vi "Channel_selector.vi"(11 "EEG_Data(all_Ch)":dbl[][](array[numeric])) -> (3 "EEG_Data(11Channel)":dbl[][](array[numeric]))   [LabVIEW 2014]
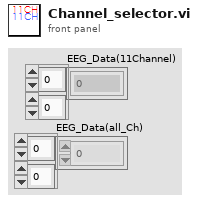
[diagram p1: front panel]
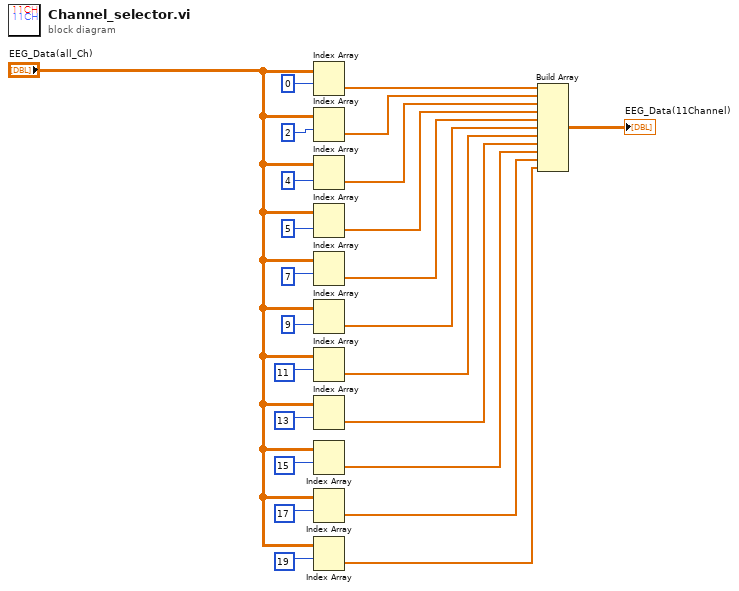
[diagram p0: block diagram]
diagram:
  n1 = Index Array(array="EEG_Data(all_Ch)", index (row)=0 ("index")) -> (element=w13:dbl[])  [unwired: 1 in]
  n2 = Index Array(array="EEG_Data(all_Ch)", index (row)=2 ("index")) -> (element=w12:dbl[])  [unwired: 1 in]
  n3 = Index Array(array="EEG_Data(all_Ch)", index (row)=4 ("index")) -> (element=w11:dbl[])  [unwired: 1 in]
  n4 = Index Array(array="EEG_Data(all_Ch)", index (row)=5 ("index")) -> (element=w10:dbl[])  [unwired: 1 in]
  n5 = Index Array(array="EEG_Data(all_Ch)", index (row)=7 ("index")) -> (element=w9:dbl[])  [unwired: 1 in]
  n6 = Index Array(array="EEG_Data(all_Ch)", index (row)=9 ("index")) -> (element=w8:dbl[])  [unwired: 1 in]
  n7 = Index Array(array="EEG_Data(all_Ch)", index (row)=11 ("index")) -> (element=w7:dbl[])  [unwired: 1 in]
  n8 = Index Array(array="EEG_Data(all_Ch)", index (row)=13 ("index")) -> (element=w6:dbl[])  [unwired: 1 in]
  n9 = Index Array(array="EEG_Data(all_Ch)", index (row)=15 ("index")) -> (element=w5:dbl[])  [unwired: 1 in]
  n10 = Index Array(array="EEG_Data(all_Ch)", index (row)=17 ("index")) -> (element=w4:dbl[])  [unwired: 1 in]
  n11 = Index Array(array="EEG_Data(all_Ch)", index (row)=19 ("index")) -> (element=w3:dbl[])  [unwired: 1 in]
  n12 = Build Array(w13, w12, w11, w10, w9, w8, w7, w6, w5, w4, w3) -> (→"EEG_Data(11Channel)":dbl[][])
